vi "Format Metric.vi"(6 "Metric Type":string, 8 "error in (no error)":errorcluster, 9 "Metric Value":dbl, 10 "Metric Name":string, 11 "StatD Interface in":refnum<class "StatD Interface.lvclass">) -> (0 "error out":errorcluster, 2 "Packet":string, 3 "StatD Interface out":refnum<class "StatD Interface.lvclass">)   [LabVIEW 2011, in "StatD Interface.lvclass"]
uses:
  StatD Interface.lvclass
panel:
  in  "Tag Values":string[](array[string])
  in  "Tags":string[](array[string])
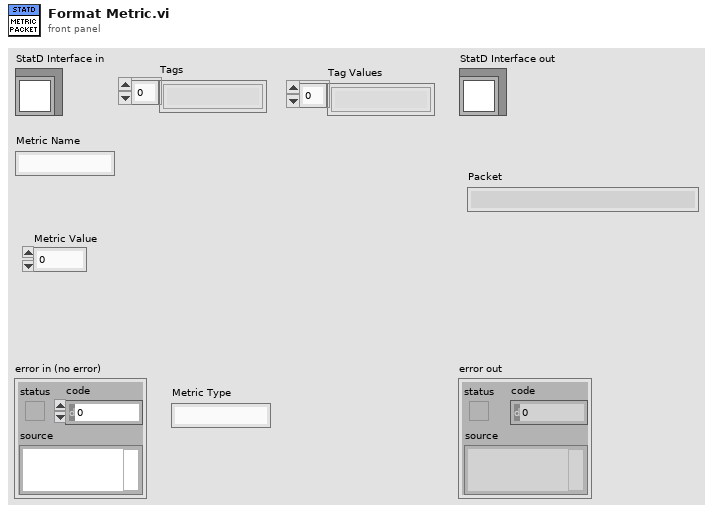
[diagram p1: front panel]
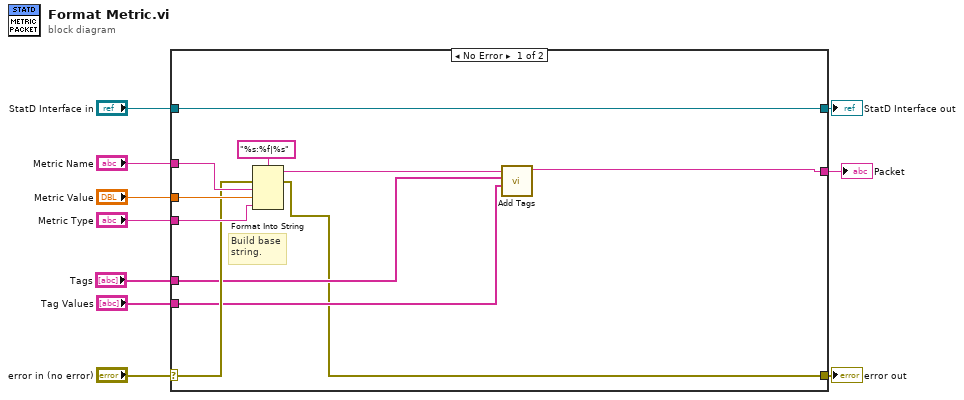
[diagram p0: block diagram]
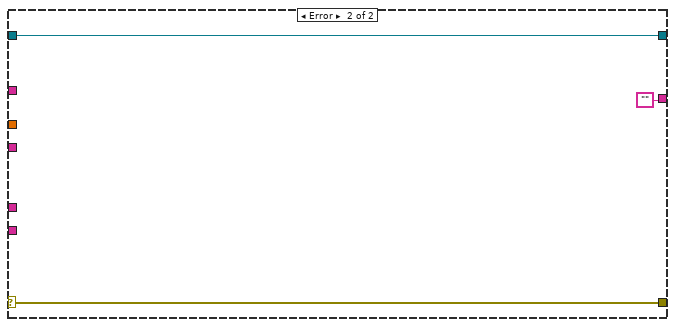
[diagram p2: hidden frame]
diagram:
  n1 = case shown="No Error" "error in (no error)" {
    selector: "error in (no error)" -> [w16 w24]
    tunnel: [w11 w24] -> w9
    tunnel: [w21 w23] -> w7
    tunnel: "StatD Interface in" -> [w21 w23]
    tunnel: "Metric Name" -> [w19 _]
    tunnel: "Metric Value" -> [w18 _]
    tunnel: "Metric Type" -> [w17 _]
    tunnel: "Tags" -> [w15 _]
    tunnel: "Tag Values" -> [w14 _]
    tunnel: [w13 ""] -> w1
    frame No Error {
      # "Build base\nstring."
      n2 = Format Into String(format string="%s:%f|%s", error in=w16, w19, w18, w17) -> (resulting string=w12:string, error out=w11:errorcluster)  [unwired: 1 in]
      n3 = call "Add Tags.vi"("Tag Values"=w14, "Tags"=w15, "Packet in"=w12) -> ("Packet out"=w13:string)  [unwired: 8 in]
    }
    frame Error {
    }
  }
  "error out" <- w9
  "StatD Interface out" <- w7
  "Packet" <- w1
